vi "Get Color Not In Image.vi"(1 "Color Array":u32[](array[numeric])) -> (0 "Color not in image":u32)   [LabVIEW 2020]
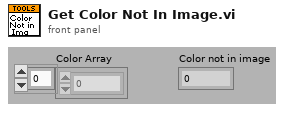
[diagram p1: front panel]
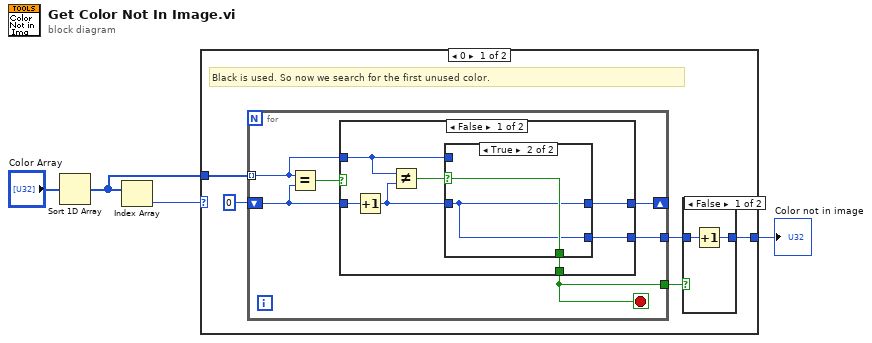
[diagram p0: block diagram]
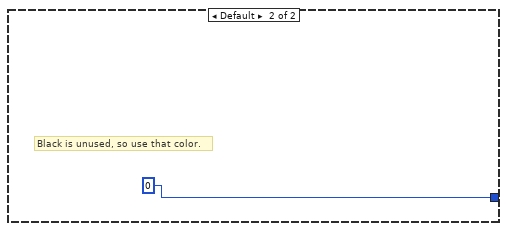
[diagram p5: hidden frame]
diagram:
  n1 = Sort 1D Array(array="Color Array") -> (sorted array=w2:u32[])
  n2 = Index Array(array=w2) -> (element=w4:u32)  [unwired: 1 in]
  n3 = case shown="0" w4 {
    tunnel: w2 -> [w9 _]
    tunnel: [w6 0] -> w1
    frame 0 {
      # "Black is used. So now we search for the first unused color."
      n4 = for {
        tunnel: w9 -> [w15] mode=indexing
        shift-right: [w16] -> _
        shift-left: u32 0 -> [w17]
        tunnel: [w14] -> w5
        tunnel: [w13] -> w7
        stop <- w13 stop-if-true
        n5 = Equal?(x=w15, y=w17) -> (x = y?=w18:bool)
        n6 = case shown="False" w18 {
          tunnel: w17 -> [w25 w29]
          tunnel: [w20 w29] -> w16
          tunnel: w15 -> [w19 _]
          tunnel: [w22 _] -> w14
          tunnel: [w21 _] -> w13
          frame False {
            n7 = Increment(x=w25) -> (x+1=w23:u32)
            n8 = Not Equal?(x=w19, y=w23) -> (x != y?=w24:bool)
            n9 = case shown="True" w24 {
              selector: w24 -> [_ w28]
              tunnel: w23 -> [_ w27]
              tunnel: [_ w27] -> w22
              tunnel: [_ w28] -> w21
              tunnel: [w26 w27] -> w20
              tunnel: w19 -> [w26 _]
              frame False {
              }
              frame True {
              }
            }
          }
          frame True {
          }
        }
      }
      n10 = case shown="False" w7 {
        tunnel: [w11 w12] -> w6
        tunnel: w5 -> [w10 w12]
        frame False {
          n11 = Increment(x=w10) -> (x+1=w11:u32)
        }
        frame True {
        }
      }
    }
    frame Default {
      # "Black is unused, so use that color."
    }
  }
  "Color not in image" <- w1
